vi "MM6.ProcDestructor.vi"(0 "i ref in":refnum<vi>, 3 "ms timeout (10000)":i32=10000, 5 "error in (no error)":errorcluster) -> (14 "i ref out":refnum<vi>, 19 "error out":errorcluster)   [LabVIEW 2014, in "MM6.lvlib"]
doc: "This is the counterpart to ProcConstructor and is called before the \"deactivate\" is called. This can be used to shutdown/deinitialize things."
uses:
  MM6.lvlib
  CS_Core/CSSystem/CoreLib/CoreLib.string 2 byte array.vi
  CS_Core/BaseProcess/BaseProcess.lvlib
  CS_Core/CSSystem/CSSystemLib/CSSystemLib.lvlib
  CS_Core/CSSystem/CoreLib/CoreLib.lvlib
  CSlibraries-extern/DimLVEvent/LVDimInterface/LVDimInterface.lvlib
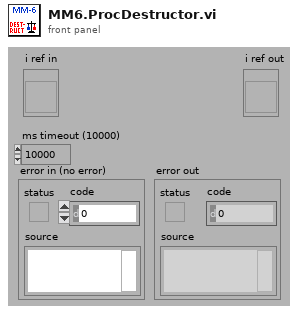
[diagram p1: front panel]
types:
  T1 = typedef "MM6.lvlib/MM6.i attribute.ctl" = cluster{"ConfigData":T2, "UsedObjs":string[], "ActScanStep":i32[], "AbortRequest":bool, "StopRequest":bool, "# cycles":i32, "Connected":bool, "MMStatus":T17, "# data":i32, "DIMServices":cluster{"MM6StatusString":string, "MM6StatusID":i32, "discArchiver":string, "discArchiverID":i32, "eventBuilder":string, "eventBuilderID":i32, "GUIIDString":string, "GUIIDStringID":i32}, "dataFile":string, "ExtraDataSets":T18, "PGRunning":T19}
  T2 = typedef "LEBITDefs.lvlib/LEBITDefs.ConfigData.ctl" = cluster{"GenConfig":T3, "Configs":T5[]}
  T3 = typedef "LEBITDefs.lvlib/LEBITDefs.GenConfig.ctl" = cluster{"Mode":i32, "Logs":T4[]}
  T4 = typedef "LEBITDefs.lvlib/LEBITDefs.Log.ctl" = cluster{"Name":string, "FctName":string, "Special":string}
  T5 = typedef "LEBITDefs.lvlib/LEBITDefs.OneConfig.ctl" = cluster{"MCA":T6, "Timing":T7, "Scans":T10[], "FreqDevs":T11[], "CleanDev":T12, "NrCycles":i32, "Specials":T14[], "Delays":T15[], "DAC":T16}
  T6 = typedef "LEBITDefs.lvlib/LEBITDefs.MCA.ctl" = cluster{"Name":string, "Address":string, "NrChannels":i32, "Gate":i32, "NrPipse":i32}
  T7 = typedef "LEBITDefs.lvlib/LEBITDefs.Timing.ctl" = cluster{"TimeTables":cluster{"TimeTable":T8}[], "Memories":T9[], "ScanX":string, "ScanY":string}
  T8 = typedef "LEBITDefs.lvlib/LEBITDefs.Timetable.ctl" = dbl[]
  T9 = typedef "LEBITDefs.lvlib/LEBITDefs.Memory.ctl" = cluster{"Device":string, "ExtTrig":bool, "TT2Use":i32, "PatternTable":string[]}
  T10 = typedef "LEBITDefs.lvlib/LEBITDefs.ScanDev.ctl" = cluster{"Name":string, "FctName":string, "Values":dbl[], "NrScanVals":i32, "Special":string}
  T11 = typedef "LEBITDefs.lvlib/LEBITDefs.FreqDev.ctl" = cluster{"Name":string, "Amp":dbl, "CenterFreq":dbl, "Time":dbl}
  T12 = typedef "LEBITDefs.lvlib/LEBITDefs.CleanDev.ctl" = cluster{"Name":string, "CleanData":T13[]}
  T13 = typedef "LEBITDefs.lvlib/LEBITDefs.CleanDataType.ctl" = cluster{"Amp":dbl, "Center":dbl, "Plus":dbl, "Minus":dbl, "Time":dbl}
  T14 = typedef "LEBITDefs.lvlib/LEBITDefs.Special.ctl" = cluster{"Name":string, "FctName":string, "VerySpecial":string, "Data":dbl}
  T15 = typedef "LEBITDefs.lvlib/LEBITDefs.Delay.ctl" = cluster{"Name":string, "Delay":dbl}
  T16 = typedef "LEBITDefs.lvlib/LEBITDefs.DAC.ctl" = cluster{"Name":string, "Step1":i32, "Step2":i32}
  T17 = typedef "MM6.lvlib/MM6.status.ctl" = enum16{"loaded", "load_error", "config", "config_error", "init", "init_error", "data_reset", "data_reset_error", "running", "start_error", "run_error", "abort_requested", "aborted", "stop_requested", "stopped", "stop_error", "Connected", "NOTConnected"}
  T18 = typedef "LEBITDefs.lvlib/LEBITDefs.ExtraData.ctl" = cluster{"Ions":cluster{"ExcitIonMass":string, "ExcitIonCharge":i32, "CleanIons":cluster{"CleanIonMass":string, "CleanIonCharge":i32}[]}, "TimingDescription":cluster{"TimeTableDescription":cluster{"Times":string[]}[], "PatternTableDescription":cluster{"Pattern":string[]}[]}, "ScanUnits":string[]}[]
  T19 = typedef "PPG_ABC.lvlib/PPG_ABC.PG_Running.ctl" = i32
  T20 = typedef "CoreDefs.rawDataType.ctl" = i8[]
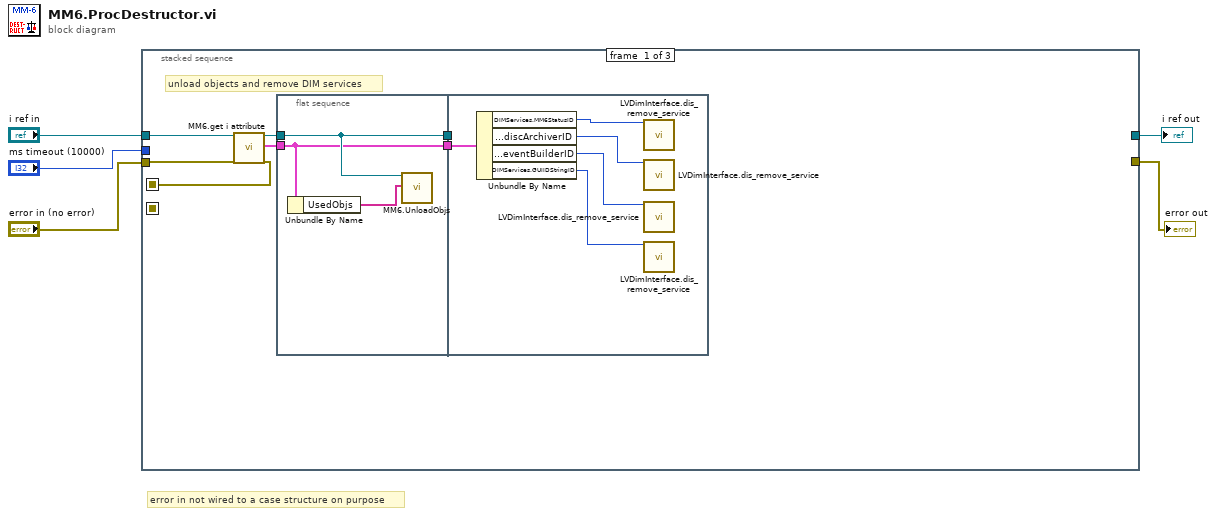
[diagram p0: block diagram]
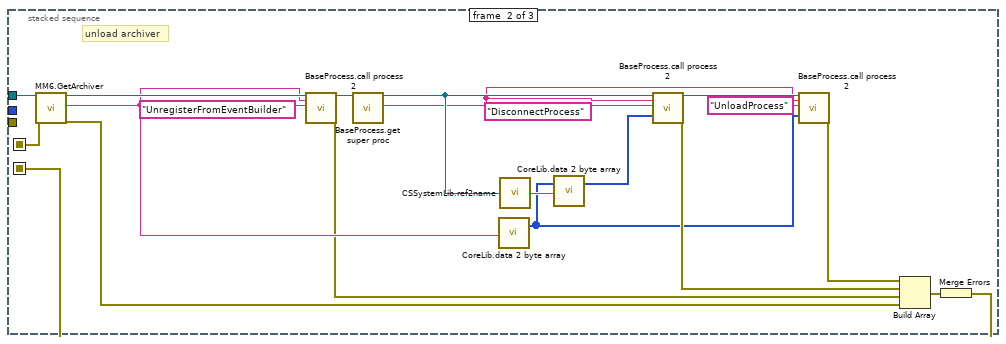
[diagram p2: hidden frame]
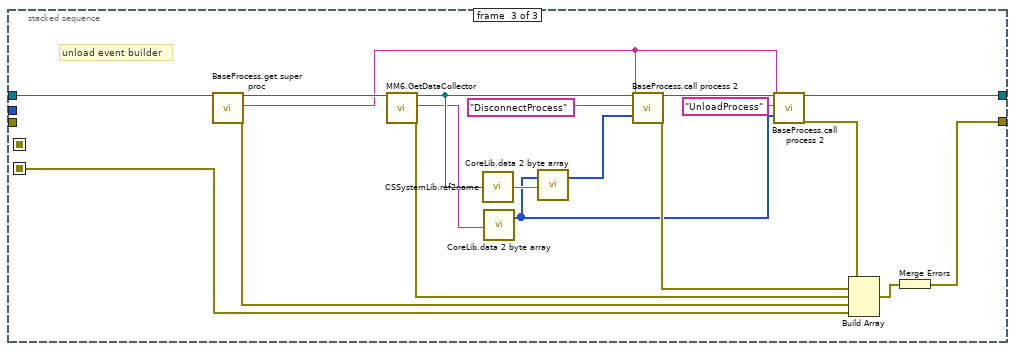
[diagram p3: hidden frame]
diagram:
  # "error in not wired to a case structure on purpose"
  n1 = stacked-sequence {
    seq-local: [_ w35 _] -> [_ _ w53]
    seq-local: [w7 _ _] -> [_ w38 _]
    tunnel: "i ref in" -> [w11 w40 w58]
    tunnel: "error in (no error)" -> [w10 _ _]
    tunnel: "ms timeout (10000)" -> [_ _ _]
    tunnel: [_ _ w41] -> w2
    tunnel: [_ _ w48] -> w1
    frame #0 {
      # "unload objects and remove DIM services"
      n2 = call "MM6.get i attribute.vi"("i ref in"=w11, "error in (no error)"=w10) -> ("i ref out"=w12:refnum<vi>, "i attribute"=w6:T1, "error out"=w7:errorcluster)  [unwired: 15 in]
      n3 = flat-sequence {
        tunnel: [w13] -> w9
        tunnel: [w14] -> w8
        tunnel: w12 -> [w14]
        tunnel: w6 -> [w13]
        tunnel: w9 -> [w20]
        tunnel: w8 -> [_]
        frame #0 {
          n4 = Unbundle By Name(w13) -> ("UsedObjs"=w15:string[])
          n5 = call "MM6.UnloadObjs.vi"("i ref in"=w14, "ObjsToUnload"=w15) -> ()  [unwired: 16 in, 2 out]
        }
        frame #1 {
          n6 = Unbundle By Name(w20) -> ("DIMServices.MM6StatusID"=w19:i32, "DIMServices.discArchiverID"=w18:i32, "DIMServices.eventBuilderID"=w17:i32, "DIMServices.GUIIDStringID"=w16:i32)
          n7 = call "LVDimInterface.dis_remove_service.vi"("my_serviceID"=w19) -> ()  [unwired: 18 in, 1 out]
          n8 = call "LVDimInterface.dis_remove_service.vi"("my_serviceID"=w18) -> ()  [unwired: 18 in, 1 out]
          n9 = call "LVDimInterface.dis_remove_service.vi"("my_serviceID"=w17) -> ()  [unwired: 18 in, 1 out]
          n10 = call "LVDimInterface.dis_remove_service.vi"("my_serviceID"=w16) -> ()  [unwired: 18 in, 1 out]
        }
      }
    }
    frame #1 {
      # "unload archiver"
      n11 = call "MM6.GetArchiver.vi"("i ref in"=w40, "error in (no error)"=w38) -> ("i ref out"=w39:refnum<vi>, "archiver"=w37:string, "error out"=w36:errorcluster)  [unwired: 15 in]
      n12 = call "BaseProcess.call process 2.vi"("i ref in"=w39, "Object"=w37, "Selector"="UnregisterFromEventBuilder") -> ("i ref out"=w34:refnum<vi>, "error out"=w28:errorcluster)  [unwired: 15 in]
      n13 = call "BaseProcess.get super proc.vi"("i ref in"=w34) -> ("i ref out"=w33:refnum<vi>, "SuperProc"=w23:string)  [unwired: 16 in, 1 out]
      n14 = call-poly "CoreLib.data 2 byte array.vi"("string"=w37) -> ("byteArray out"=w21:T20)  [unwired: 18 in]
      n15 = call "CSSystemLib.ref2name.vi"("obj refnum"=w33) -> ("name"=w30:string)
      n16 = call-poly "CoreLib.data 2 byte array.vi"("byteArray"=w21, "string"=w30) -> ("byteArray out"=w29:T20)  [unwired: 17 in]
      n17 = call "BaseProcess.call process 2.vi"("i ref in"=w33, "Object"=w23, "Selector"="DisconnectProcess", "Data"=w29) -> ("i ref out"=w24:refnum<vi>, "error out"=w26:errorcluster)  [unwired: 14 in]
      n18 = call "BaseProcess.call process 2.vi"("i ref in"=w24, "Object"=w23, "Selector"="UnloadProcess", "Data"=w21) -> ("error out"=w25:errorcluster)  [unwired: 14 in, 1 out]
      n19 = Build Array(w25, w26, w28, w36) -> (w27:errorcluster[])
      n20 = Merge Errors(w27) -> (w35:errorcluster)
    }
    frame #2 {
      # "unload event builder"
      n21 = call "BaseProcess.get super proc.vi"("i ref in"=w58) -> ("i ref out"=w59:refnum<vi>, "SuperProc"=w45:string, "error out"=w52:errorcluster)  [unwired: 16 in]
      n22 = call "MM6.GetDataCollector.vi"("i ref in"=w59) -> ("i ref out"=w57:refnum<vi>, "data collector"=w47:string, "error out"=w51:errorcluster)  [unwired: 16 in]
      n23 = call "CSSystemLib.ref2name.vi"("obj refnum"=w57) -> ("name"=w55:string)
      n24 = call-poly "CoreLib.data 2 byte array.vi"("string"=w47) -> ("byteArray out"=w42:T20)  [unwired: 18 in]
      n25 = call-poly "CoreLib.data 2 byte array.vi"("byteArray"=w42, "string"=w55) -> ("byteArray out"=w54:T20)  [unwired: 17 in]
      n26 = call "BaseProcess.call process 2.vi"("i ref in"=w57, "Object"=w45, "Selector"="DisconnectProcess", "Data"=w54) -> ("i ref out"=w46:refnum<vi>, "error out"=w50:errorcluster)  [unwired: 14 in]
      n27 = call "BaseProcess.call process 2.vi"("i ref in"=w46, "Object"=w45, "Selector"="UnloadProcess", "Data"=w42) -> ("i ref out"=w41:refnum<vi>, "error out"=w43:errorcluster)  [unwired: 14 in]
      n28 = Build Array(w43, w50, w51, w52, w53) -> (w49:errorcluster[])
      n29 = Merge Errors(w49) -> (w48:errorcluster)
    }
  }
  "error out" <- w1
  "i ref out" <- w2
